vi "Copy cRIO DLLs.vi"(8 "error in":errorcluster) -> (0 "error out":errorcluster)   [LabVIEW 2021, in "SEECD System Explorer.lvlib"]
uses:
  SEECD System Explorer.lvlib
  <vilib>/Utility/sysdir.llb/Get System Directory.vi
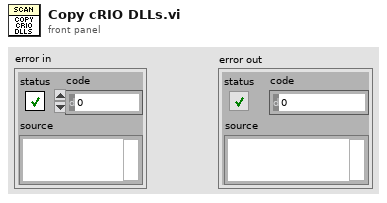
[diagram p1: front panel]
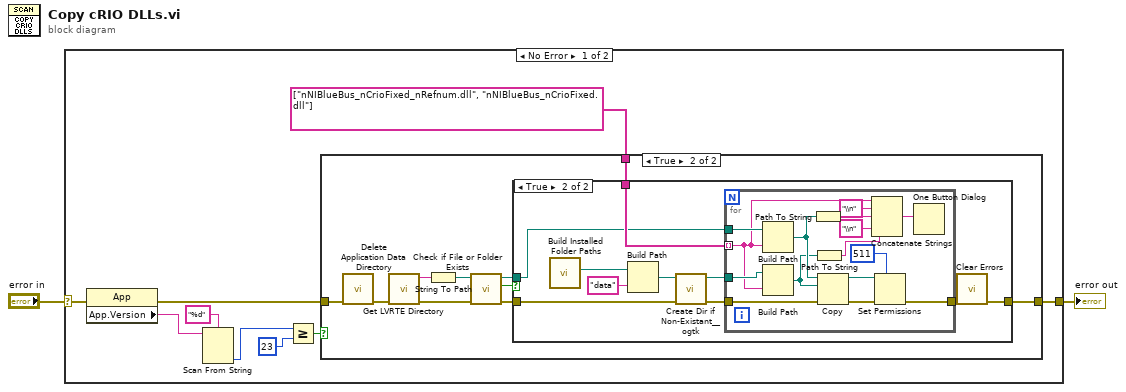
[diagram p0: block diagram]
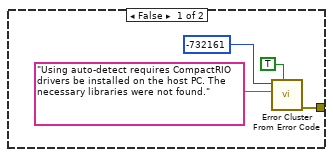
[diagram p3: hidden frame]
diagram:
  n1 = case shown="No Error" "error in" {
    selector: "error in" -> [w11 w52]
    tunnel: [w7 w52] -> w1
    frame No Error {
      n2 = property class="App"(error in=w11) -> (error out=w8:errorcluster, "App.Version"=w5:string)  [unwired: 1 in, 1 out]
      n3 = Scan From String(format string="%d", input string=w5) -> (output 1=w3:i32)  [unwired: 3 in, 3 out]
      n4 = Greater Or Equal?(x=w3, y=23) -> (x >= y?=w9:bool)
      n5 = case shown="True" w9 {
        tunnel: w8 -> [w12 w22]
        tunnel: [w12 w19] -> w7
        tunnel: string[] ["nNIBlueBus_nCrioFixed_nRefnum.dll", "nNIBlueBus_nCrioFixed.dll"] -> [_ w17]
        frame False {
        }
        frame True {
          n6 = call "Delete Application Data Directory.vi"("error in"=w22) -> ("error out"=w16:errorcluster)  [unwired: 10 in]
          n7 = call "Get LVRTE Directory.vi"("error in"=w16) -> ("error out"=w15:errorcluster, "LVRTE 2022 Directory"=w14:string)  [unwired: 9 in]
          n8 = String To Path(string=w14) -> (path=w13:path)
          n9 = call <vilib>:"Check if File or Folder Exists.vi"("error in (no error)"=w15, "path"=w13) -> ("error out"=w21:errorcluster, "file or folder exists?"=w20:bool, "dup path"=w18:path)  [unwired: 7 in]
          n10 = case shown="True" w20 {
            tunnel: w21 -> [_ w32]
            tunnel: [w23 w27] -> w19
            tunnel: w18 -> [_ w35]
            tunnel: w17 -> [_ w36]
            frame False {
              n11 = call <vilib>:"Error Cluster From Error Code.vi"("show call chain? (False)"=TRUE, "error message (\"\")"="Using auto-detect requires CompactRIO drivers be installed on the host PC. The necessary libraries were not found." ("source"), "error code (0)"=-732161 ("code")) -> ("error out"=w23:errorcluster)  [unwired: 6 in]
            }
            frame True {
              n12 = call "Build Installed Folder Paths.vi"() -> ("Application Folder Path"=w34:path)  [unwired: 10 in, 1 out]
              n13 = Build Path(base path=w34, name or relative path="data") -> (appended path=w31:path)
              n14 = call <userlib>:"Create Dir if Non-Existant__ogtk.vi"("error in (no error)"=w32, "Directory Path"=w31) -> ("error out"=w29:errorcluster, "dup Directory Path"=w30:path)  [unwired: 7 in, 1 out]
              n15 = for {
                tunnel: w36 -> [w42] mode=indexing
                tunnel: w35 -> [w51]
                tunnel: w30 -> [w49]
                tunnel: w29 -> [w50]
                tunnel: [w47] -> w28
                n16 = Build Path(base path=w51, name or relative path=w42) -> (appended path=w43:path)
                n17 = Build Path(base path=w49, name or relative path=w42) -> (appended path=w38:path)
                n18 = Path To String(path=w43) -> (string=w40:string)
                n19 = Path To String(path=w38) -> (string=w37:string)
                n20 = Copy(8:w50, 10:w38, 11:w43) -> (0:w48:errorcluster, 3:w46:path)  [unwired: 2 in, 1 out]
                n21 = Concatenate Strings(w42, "\\n" ("string"), w40, "\\n" ("string"), w37) -> (w44:string)
                n22 = Set Permissions(7:i16 511 ("permissions"), 8:w48, 11:w46) -> (0:w47:errorcluster)  [unwired: 2 in, 1 out]
                n23 = One Button Dialog(message=w44) -> ()  [unwired: 1 in, 1 out]
              }
              n24 = call <vilib>:"Clear Errors.vi"("error in (no error)"=w28) -> ("error out"=w27:errorcluster)  [unwired: 5 in, 1 out]
            }
          }
        }
      }
    }
    frame Error {
    }
  }
  "error out" <- w1
